vi "Set Variable.vi"(8 "error in (no error)":errorcluster, 9 "Value":variant, 10 "Name":string, 11 "Project in":refnum<class "Project.lvclass">) -> (0 "error out":errorcluster, 3 "Project out":refnum<class "Project.lvclass">)   [LabVIEW 2015, in "Project.lvclass"]
uses:
  Project.lvclass
  <vilib>/Utility/error.llb/Error Cluster From Error Code.vi
  <vilib>/ErrorRing/Error Ring.xnode
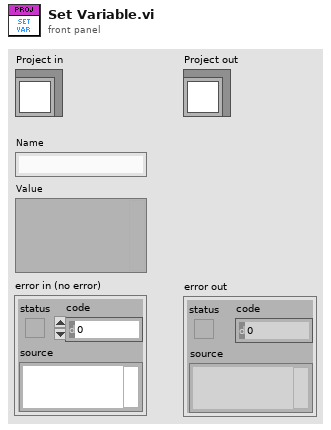
[diagram p1: front panel]
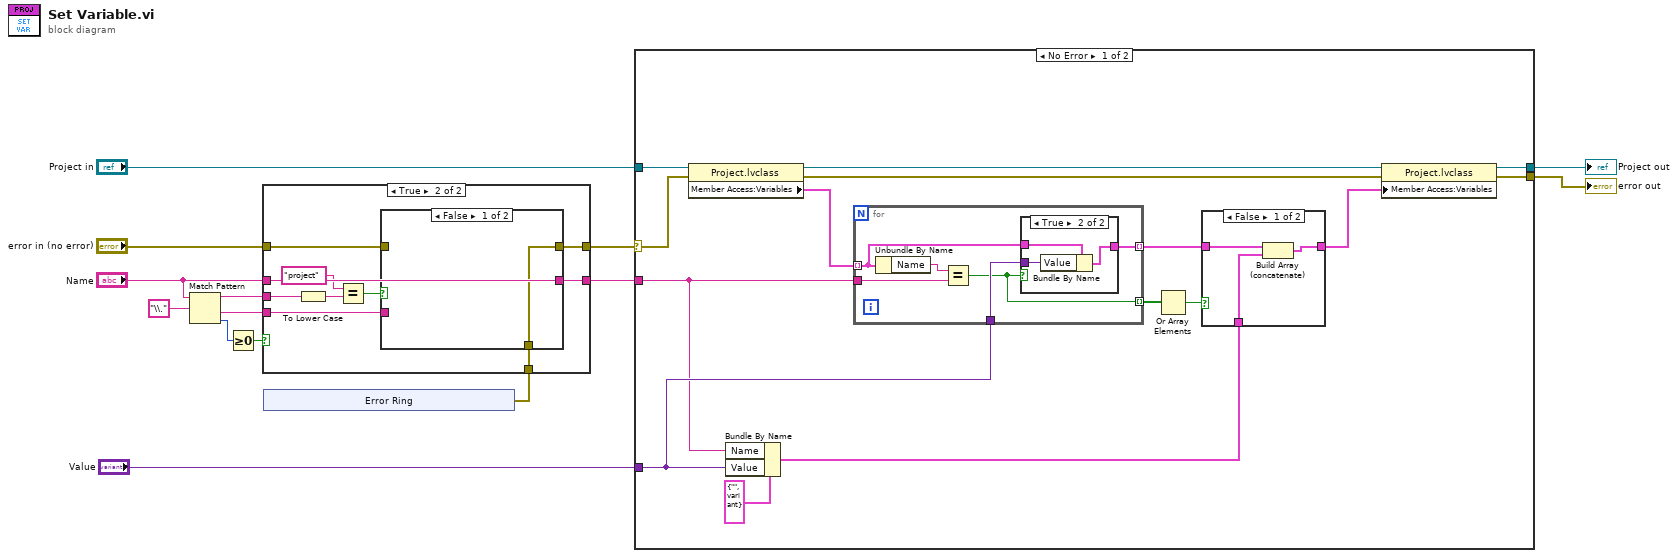
[diagram p0: block diagram]
diagram:
  n1 = Match Pattern(string="Name", regular expression="\\.") -> (before substring=w4:string, after substring=w5:string, offset past match=w8:i32)  [unwired: 1 in, 1 out]
  n2 = Greater Or Equal To 0?(x=w8) -> (x >= 0?=w7:bool)
  n3 = xnode "Error Ring"() -> ("error out"=w2:errorcluster)
  n4 = case shown="True" w7 {
    tunnel: "Name" -> [w15 _]
    tunnel: w5 -> [_ w20]
    tunnel: [w15 w19] -> _
    tunnel: w4 -> [_ w24]
    tunnel: "error in (no error)" -> [w14 w18]
    tunnel: w2 -> [_ w17]
    tunnel: [w14 w16] -> w1
    frame False {
    }
    frame True {
      n5 = To Lower Case(string=w24) -> (all lower case string=w23:string)
      n6 = Equal?(x="project", y=w23) -> (x = y?=w21:bool)
      n7 = case shown="False" w21 {
        tunnel: w20 -> [_ w27]
        tunnel: [_ w27] -> w19
        tunnel: w18 -> [_ w26]
        tunnel: w17 -> [w25 _]
        tunnel: [w25 w26] -> w16
        frame False {
        }
        frame True {
        }
      }
    }
  }
  n8 = case shown="No Error" w1 {
    selector: w1 -> [w28 w58]
    tunnel: "Project in" -> [w39 w57]
    tunnel: "Value" -> [w35 _]
    tunnel: [w31 w57] -> w11
    tunnel: [w30 w58] -> w10
    tunnel: "Name" -> [w29 _]
    frame No Error {
      n9 = property class="Project.lvclass"(reference=w39, error in=w28) -> (reference out=w34:refnum<class "Project.lvclass">, error out=w33:errorcluster, "Member Access:Variables"=w38:cluster{"Name":string, "Value":variant}[])
      n10 = Bundle By Name(cluster=cluster{"Name":string, "Value":variant} {"Name"="", "Value"=variant} ("Variable"), "Name"=w29, "Value"=w35) -> (w36:cluster{"Name":string, "Value":variant})
      n11 = for {
        tunnel: w29 -> [w51]
        tunnel: w38 -> [w50] mode=indexing
        tunnel: w35 -> [w49]
        tunnel: [w48] -> w40 mode=indexing
        tunnel: [w47] -> w42 mode=indexing
        n12 = Unbundle By Name(w50) -> ("Name"=w52:string)
        n13 = Equal?(x=w52, y=w51) -> (x = y?=w47:bool)
        n14 = case shown="True" w47 {
          tunnel: w50 -> [w53 w56]
          tunnel: w49 -> [_ w55]
          tunnel: [w53 w54] -> w48
          frame False {
          }
          frame True {
            n15 = Bundle By Name(cluster=w56, "Value"=w55) -> (w54:cluster{"Name":string, "Value":variant})
          }
        }
      }
      n16 = Or Array Elements(Boolean array=w42) -> (logical OR=w41:bool)
      n17 = case shown="False" w41 {
        tunnel: w40 -> [w45 w46]
        tunnel: w36 -> [w44 _]
        tunnel: [w43 w46] -> w32
        frame False {
          n18 = Build Array (concatenate)(w45, w44) -> (w43:cluster{"Name":string, "Value":variant}[])
        }
        frame True {
        }
      }
      n19 = property class="Project.lvclass"(reference=w34, error in=w33, "Member Access:Variables"=w32) -> (reference out=w31:refnum<class "Project.lvclass">, error out=w30:errorcluster)
    }
    frame Error {
    }
  }
  "error out" <- w10
  "Project out" <- w11
